vi "_Config Updated.vi"(8 "error in (no error)":errorcluster, 10 "Config Map":map{string, string}(c390), 11 "DeployTCPResource in":refnum<class "TCPResource.lvclass">) -> (0 "error out":errorcluster, 3 "DeployTCPResource out":refnum<class "TCPResource.lvclass">)   [LabVIEW 2020, in "PicoG-Core.lvlib" / "TCPResource.lvclass"]
uses:
  TCPResource.lvclass
  TCPResource.lvclass/TCPResource.ctl
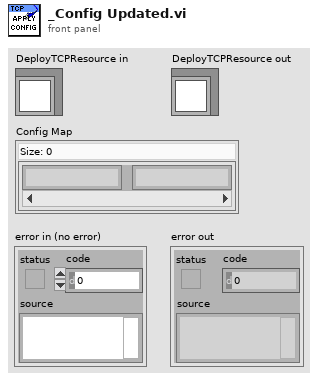
[diagram p1: front panel]
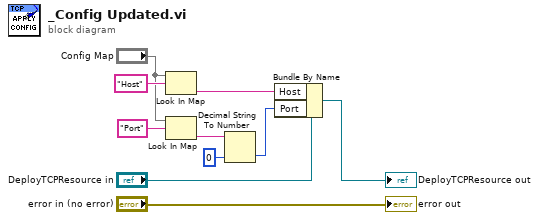
[diagram p0: block diagram]
diagram:
  n1 = Look In Map(map="Config Map", key="Host") -> (value=w4:string)  [unwired: 1 in, 1 out]
  n2 = Look In Map(map="Config Map", key="Port") -> (value=w6:string)  [unwired: 1 in, 1 out]
  n3 = Decimal String To Number(string=w6, default (0L)=u16 0 ("default (0 I32)")) -> (number=w3:u16)  [unwired: 1 in, 1 out]
  n4 = Bundle By Name(cluster="DeployTCPResource in", "Host"=w4, "Port"=w3) -> (→"DeployTCPResource out":refnum<class "TCPResource.lvclass">)
  "error out" <- "error in (no error)"
